vi "Get CAN Database Settings.vi"(8 "error in (no error)":errorcluster, 10 "Frames":cluster{"Frame":string, "Signals":string[]}[](array[cluster]), 11 "Database":string) -> (0 "error out":errorcluster, 2 "Frames":T1[](array[typedef]))   [LabVIEW 2019, in "Simple SysDef API.lvlib"]
uses:
  <userlib>/SimpleSysDef/Simple SysDef API.lvlib
  <userlib>/SimpleSysDef/_SubVIs/Add NI-XNET CAN Hardware_Frame Settings.ctl
  <userlib>/SimpleSysDef/_SubVIs/Add NI-XNET CAN Hardware_Signal Settings.ctl
  <vilib>/xnet/xnet.llb/XNET Database Open (Frame).vi
  <vilib>/xnet/xnet.llb/XNET Database Close (Frame).vi
  <vilib>/xnet/xnet.llb/XNET Database Open (Signal).vi
  <vilib>/xnet/xnet.llb/XNET Database Close (Signal).vi
  <resource>/objmgr/xnet.rc
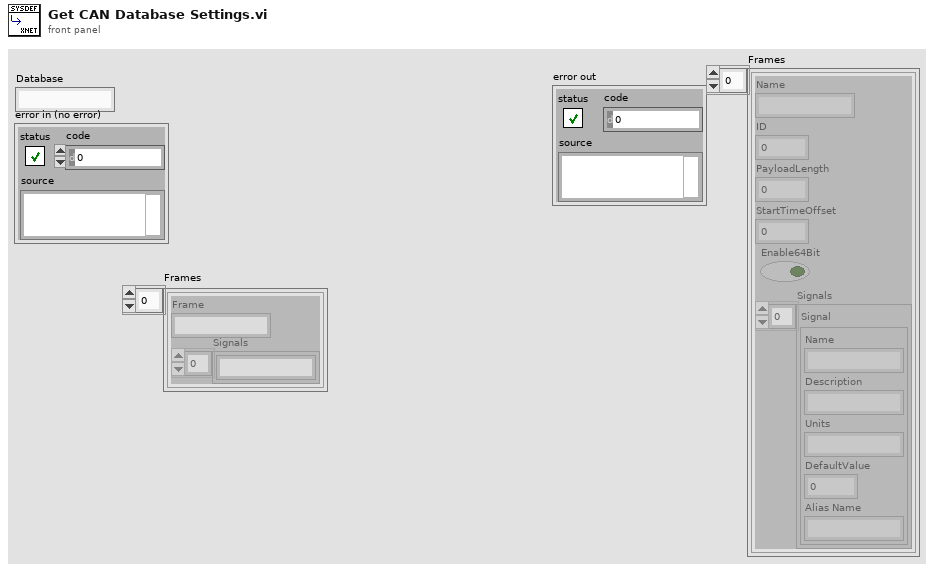
[diagram p1: front panel]
types:
  T1 = typedef "Simple SysDef API.lvlib/Add NI-XNET CAN Hardware_Frame Settings.ctl" = cluster{"Name":string, "ID":u32, "PayloadLength":u32, "StartTimeOffset":dbl, "Enable64Bit":bool, "Signals":T2[]}
  T2 = typedef "Simple SysDef API.lvlib/Add NI-XNET CAN Hardware_Signal Settings.ctl" = cluster{"Name":string, "Description":string, "Units":string, "DefaultValue":dbl, "Alias Name":string}
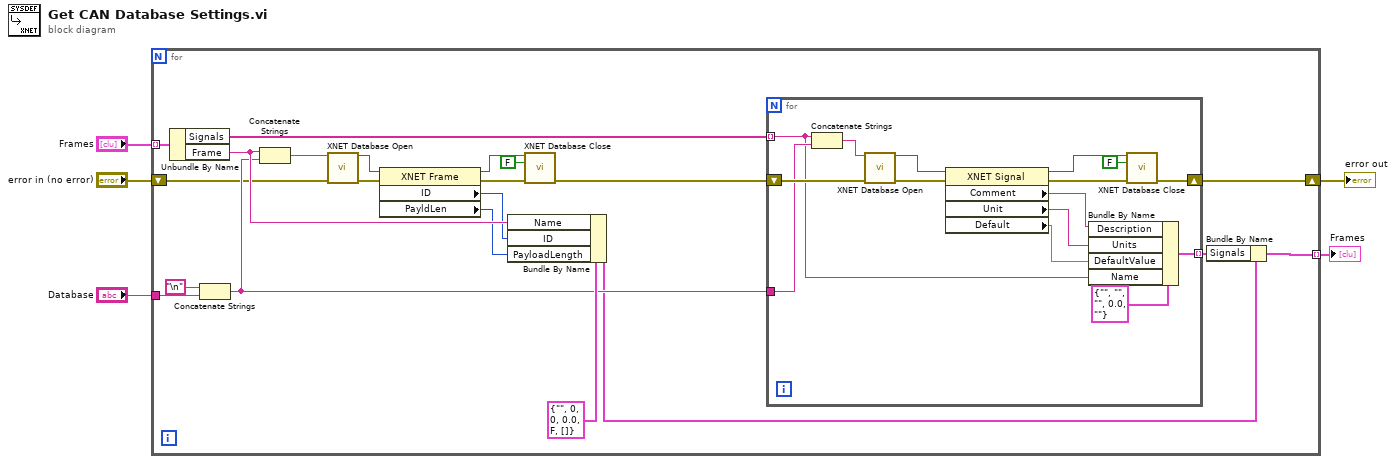
[diagram p0: block diagram]
diagram:
  n1 = for {
    tunnel: "Frames" -> [w20] mode=indexing
    tunnel: "Database" -> [w18]
    tunnel: [w8] -> w1 mode=indexing
    shift-right: [w7] -> w3
    shift-left: "error in (no error)" -> [w6]
    n2 = Unbundle By Name(w20) -> ("Signals"=w12:string[], "Frame"=w15:string)
    n3 = Concatenate Strings("\n", w18) -> (w11:string)
    n4 = Concatenate Strings(w15, w11) -> (w17:string)
    n5 = call-poly <vilib>:"XNET Database Open.vi"("frame in"=w17, "error in (no error)"=w6) -> ("frame out"=w26:refnum<k21>, "error out"=w23:errorcluster)  [unwired: 12 in]
    n6 = property class="XNET Frame"(reference=w26, error in=w23) -> (reference out=w25:refnum<k21>, error out=w24:errorcluster, "ID"=w14:u32, "PayldLen"=w13:u32)
    n7 = Bundle By Name(cluster=T1 {"Name"="", "ID"=0, "PayloadLength"=0, "StartTimeOffset"=0.0, "Enable64Bit"=FALSE, "Signals"=[]} ("Frame Settings"), "Name"=w15, "ID"=w14, "PayloadLength"=w13) -> (w10:T1)
    n8 = call-poly <vilib>:"XNET Database Close.vi"("frame in"=w25, "close all? (true)"=FALSE, "error in (no error)"=w24) -> ("error out"=w22:errorcluster)  [unwired: 12 in]
    n9 = for {
      shift-right: [w35] -> w7
      shift-left: w22 -> [w41]
      tunnel: w12 -> [w31] mode=indexing
      tunnel: w11 -> [w34]
      tunnel: [w27] -> w9 mode=indexing
      n10 = Concatenate Strings(w31, w34) -> (w33:string)
      n11 = call-poly <vilib>:"XNET Database Open.vi"("signal in"=w33, "error in (no error)"=w41) -> ("signal out"=w39:refnum<k21>, "error out"=w40:errorcluster)  [unwired: 12 in]
      n12 = property class="XNET Signal"(reference=w39, error in=w40) -> (reference out=w36:refnum<k21>, error out=w37:errorcluster, "Comment"=w30:string, "Unit"=w29:string, "Default"=w28:dbl)
      n13 = Bundle By Name(cluster=T2 {"Name"="", "Description"="", "Units"="", "DefaultValue"=0.0, "Alias Name"=""} ("Signal"), "Description"=w30, "Units"=w29, "DefaultValue"=w28, "Name"=w31) -> (w27:T2)
      n14 = call-poly <vilib>:"XNET Database Close.vi"("signal in"=w36, "close all? (true)"=FALSE, "error in (no error)"=w37) -> ("error out"=w35:errorcluster)  [unwired: 12 in]
    }
    n15 = Bundle By Name(cluster=w10, "Signals"=w9) -> (w8:T1)
  }
  "error out" <- w3
  "Frames" <- w1
